vi "Lookup APIs of Type.vi"(8 "error in (no error)":errorcluster, 11 "Task in":refnum<class "Task.lvclass">) -> (0 "error out":errorcluster, 3 "Task out":refnum<class "Task.lvclass">)   [LabVIEW 2020, in "Volatus.lvlib" / "Task.lvclass"]
uses:
  Task.lvclass
  Identity/Identity.lvclass
  API/API.lvclass
  Task.lvclass/Task.ctl
  VolatusAPI/VolatusAPI.lvclass/VolatusAPI.ctl
  VolatusAPI/VolatusAPI.lvclass
panel:
  out "APIs":refnum<class "API.lvclass">[](array[class])
  in  "Identity - Type Only":refnum<class "Identity.lvclass">
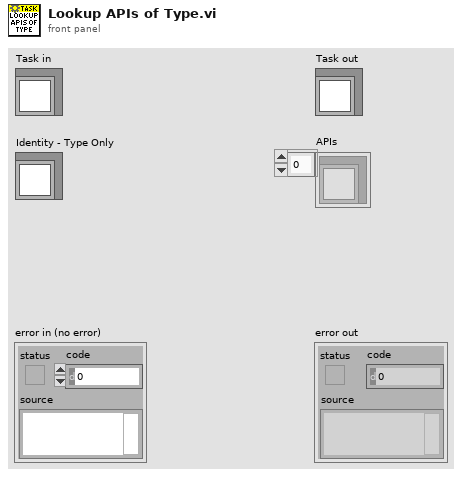
[diagram p1: front panel]
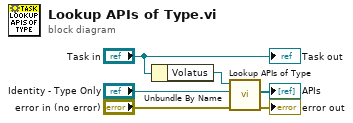
[diagram p0: block diagram]
diagram:
  n1 = Unbundle By Name("Task in") -> ("Volatus"=w5:refnum<class "VolatusAPI.lvclass">)
  n2 = call "Lookup APIs of Type.vi"("error in (no error)"="error in (no error)", "Identity - Type Only"="Identity - Type Only", "VolatusAPI in"=w5) -> ("error out"=→"error out":errorcluster, "APIs"=→"APIs":refnum<class "API.lvclass">[])  [unwired: 6 in, 1 out]
  "Task out" <- "Task in"
